vi "ScaleAI16_src.vi"(0 "UnscaledAI":i16[](array[numeric])=[0, 0, 0, 0, 0, 0, 0, 0, 0, 0, 0, 0, 0, 0, 0, 0], 7 "B":i16[](array[numeric])=[0, 0, 0, 0, 0, 0, 0, 0, 0, 0, 0, 0, 0, 0, 0, 0], 9 "M":sgl[](array[numeric])=[0.0, 0.0, 0.0, 0.0, 0.0, 0.0, 0.0, 0.0, 0.0, 0.0, 0.0, 0.0, 0.0, 0.0, 0.0, 0.0]) -> (4 "ScaledAI":sgl[](array[numeric]))   [LabVIEW 2017]
doc: "Scales U32 to SGL data type. Based on Y=M*(X-B)"
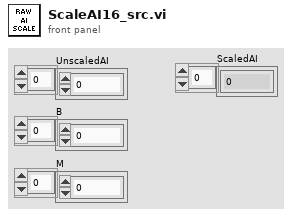
[diagram p1: front panel]
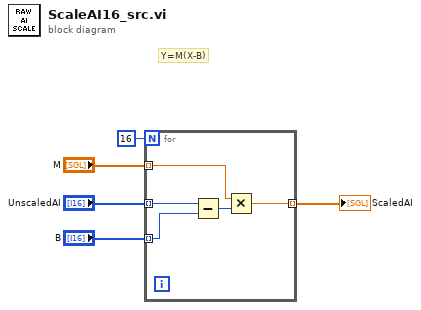
[diagram p0: block diagram]
diagram:
  # "Y=M(X-B)"
  n1 = for {
    N: 16 -> [_]
    tunnel: "UnscaledAI" -> [w10] mode=indexing
    tunnel: "B" -> [w9] mode=indexing
    tunnel: "M" -> [w7] mode=indexing
    tunnel: [w6] -> w2 mode=indexing
    n2 = Subtract(x=w10, y=w9) -> (x-y=w8:i16)
    n3 = Multiply(x=w7, y=w8) -> (x*y=w6:sgl)
  }
  "ScaledAI" <- w2
